vi "write_syncout_command.vi"(11 "SYNC Output":T1(ring)) -> (3 "Command Out":string)   [LabVIEW 2015]
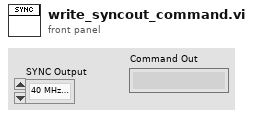
[diagram p1: front panel]
types:
  T1 = enum16{"40 MHz Clock", "Gate Disc Signal", "Trigger Disc Signal", "Counter 1 Disc Signal", "Counter 2 Disc Signal", "Definitely Not Used", "Not Used", "1 kHz Signal", "Also Not Used", "MCS On/Off", "End of Time Bin", "Ramp Increment Trig", "Step Count Trigger", "'GO'-Line", "Ramp Down Trigger", "Logic 1"}
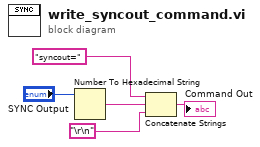
[diagram p0: block diagram]
diagram:
  n1 = Number To Hexadecimal String(2:"SYNC Output") -> (0:w3:string)  [unwired: 1 in]
  n2 = Concatenate Strings("syncout=" ("string"), w3, "\r\n") -> (→"Command Out":string)
